vi "PalmSense Configure Time.vi"(8 "error in (no error)":errorcluster, 10 "Message Data":variant, 11 "Data Cluster in":T1) -> (0 "error out":errorcluster, 2 "Send Resp":bool, 3 "Data Cluster out":T1)   [LabVIEW 2020, in "PalmSens.lvlib"]
uses:
  PalmSens.lvlib
  PalmSense Hardware Configuration.ctl
  <instrlib>/PalmSens SDK for LabVIEW 5.10/PalmSens/PalmSens.lvclass
  support/Message Queue/Message Cluster.ctl
  support/HW Message Cluster.ctl
  support/Message Queue/Message Queue.lvlib
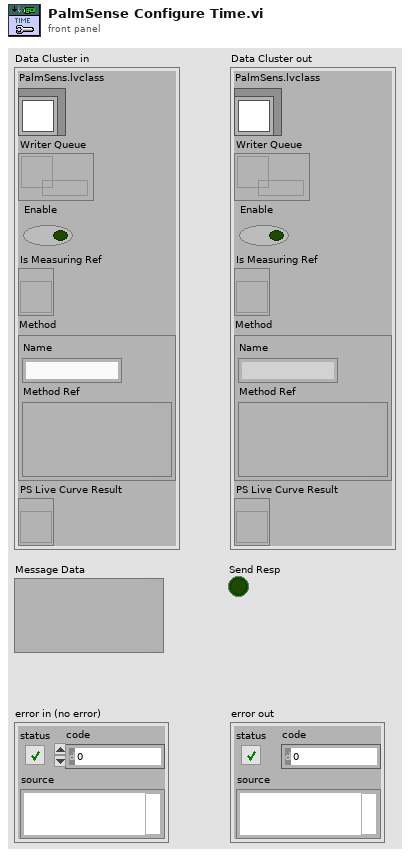
[diagram p1: front panel]
types:
  T1 = typedef "PalmSens.lvlib/PalmSense Hardware Configuration.ctl" = cluster{"PalmSens.lvclass":refnum<class "PalmSens.lvclass">, "Writer Queue":refnum<queue>, "Enable":bool, "Is Measuring Ref":refnum<vi>, "Method":cluster{"Name":string, "Method Ref":variant}, "PS Live Curve Result":refnum<vi>}
  T2 = typedef "Message Queue.lvlib/HW Message Cluster.ctl" = cluster{"Writer Queue":refnum<queue>, "Writer Data":T3}
  T3 = typedef "Message Queue.lvlib/Message Cluster.ctl" = cluster{"Message":string, "Message Data":variant}
  T4 = cluster{"Timebase (0.0005 s)":dbl, "Position (0.0 s)":dbl}
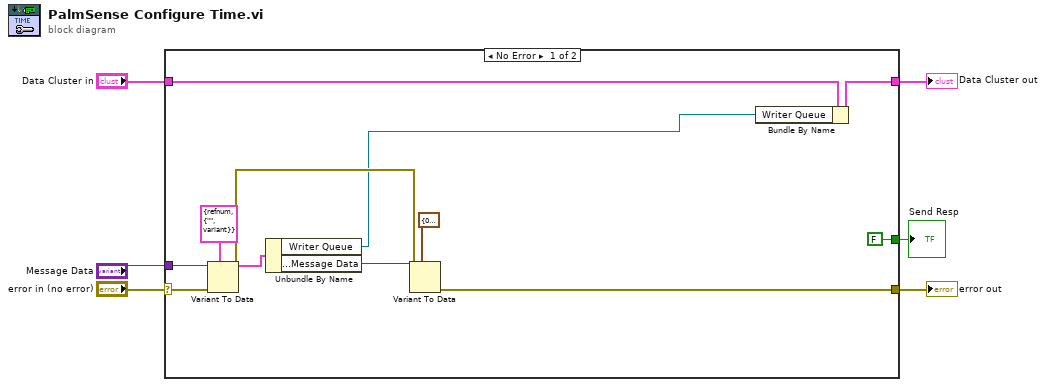
[diagram p0: block diagram]
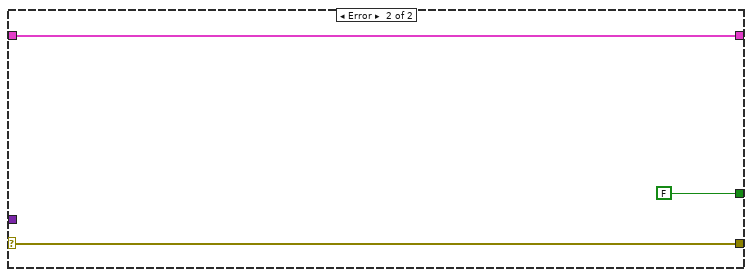
[diagram p2: hidden frame]
diagram:
  n1 = case shown="No Error" "error in (no error)" {
    selector: "error in (no error)" -> [w12 w21]
    tunnel: "Message Data" -> [w13 _]
    tunnel: [w18 w20] -> w5
    tunnel: "Data Cluster in" -> [w17 w20]
    tunnel: [w9 w21] -> w3
    tunnel: [FALSE ("Send Resp") FALSE ("Send Resp")] -> w1
    frame No Error {
      n2 = Variant To Data(error in=w12, type=T2 {"Writer Queue"=refnum, "Writer Data"={"Message"="", "Message Data"=variant}}, Variant=w13) -> (data=w14:T2, error out=w11:errorcluster)
      n3 = Unbundle By Name(w14) -> ("Writer Queue"=w8:refnum<queue>, "Writer Data.Message Data"=w7:variant)
      n4 = Variant To Data(error in=w11, type=T4 {"Timebase (0.0005 s)"=0.0005, "Position (0.0 s)"=0.0}, Variant=w7) -> (error out=w9:errorcluster)  [unwired: 1 out]
      n5 = Bundle By Name(cluster=w17, "Writer Queue"=w8) -> (w18:T1)
    }
    frame Error {
    }
  }
  "Data Cluster out" <- w5
  "error out" <- w3
  "Send Resp" <- w1
